vi "Initialize Editor Handler.vi"(8 "error in (no error)":errorcluster, 9 "Clear Picture?":bool=TRUE, 10 "PictureRef":refnum<vi>, 11 "Editor Handler in":refnum<class "Image Editor Handler.lvclass">) -> (0 "error out":errorcluster, 3 "Editor Handler out":refnum<class "Image Editor Handler.lvclass">)   [LabVIEW 2015, in "LV Image Editor Framework.lvlib" / "Image Editor Handler.lvclass"]
uses:
  Image Editor Handler.lvclass
  Image Editor Handler.lvclass/Image Editor Handler.ctl
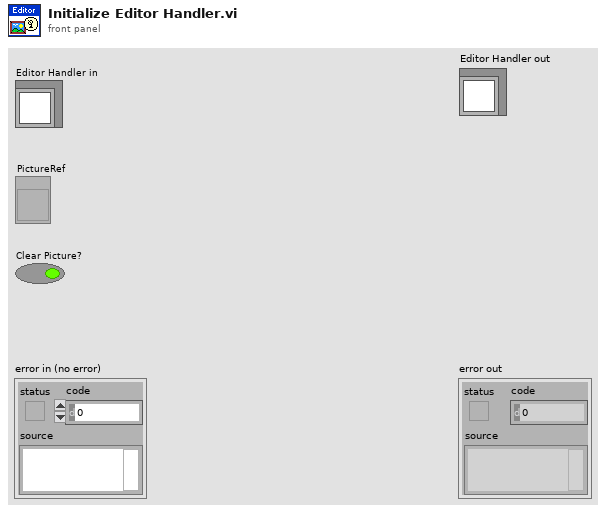
[diagram p1: front panel]
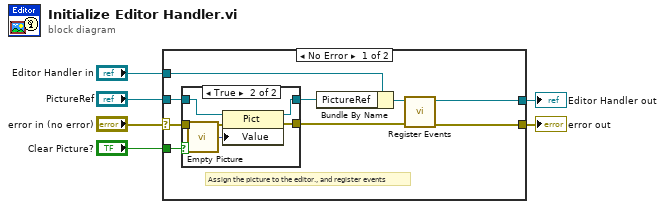
[diagram p0: block diagram]
diagram:
  n1 = case shown="No Error" "error in (no error)" {
    selector: "error in (no error)" -> [w12 w24]
    tunnel: [w13 w24] -> w6
    tunnel: [w7 w23] -> w4
    tunnel: "Editor Handler in" -> [w15 w23]
    tunnel: "PictureRef" -> [w10 _]
    tunnel: "Clear Picture?" -> [w8 _]
    frame No Error {
      # "Assign the picture to the editor., and register events"
      n2 = case shown="True" w8 {
        tunnel: w12 -> [w16 w22]
        tunnel: [w16 w21] -> w11
        tunnel: w10 -> [w17 w20]
        tunnel: [w17 w19] -> w9
        frame False {
        }
        frame True {
          n3 = call "Empty Picture"() -> ("empty picture"=w18:picture)
          n4 = property class="Pict"(reference=w20, error in=w22, "Value"=w18) -> (reference out=w19:refnum<vi>, error out=w21:errorcluster)
        }
      }
      n5 = Bundle By Name(cluster=w15, "PictureRef"=w9) -> (w14:refnum<class "Image Editor Handler.lvclass">)
      n6 = call-dynamic "Register Events.vi"("error in (no error)"=w11, "Editor Handler in"=w14) -> ("error out"=w13:errorcluster, "Editor Handler out"=w7:refnum<class "Image Editor Handler.lvclass">)  [unwired: 8 in]
    }
    frame Error {
    }
  }
  "error out" <- w6
  "Editor Handler out" <- w4
